vi "readAtom.vi"(4 "error in":errorcluster, 7 "Byte Stream File":refnum<file>) -> (0 "error out":errorcluster, 1 "String":string, 3 "Byte Stream File Refnum":refnum<file>)   [LabVIEW 2010]
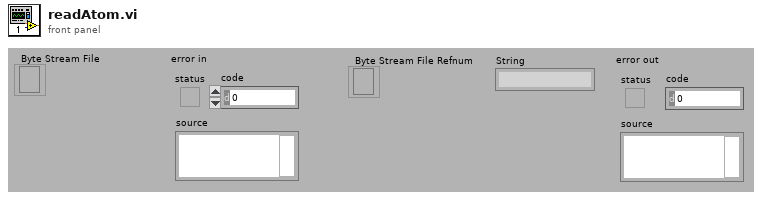
[diagram p1: front panel]
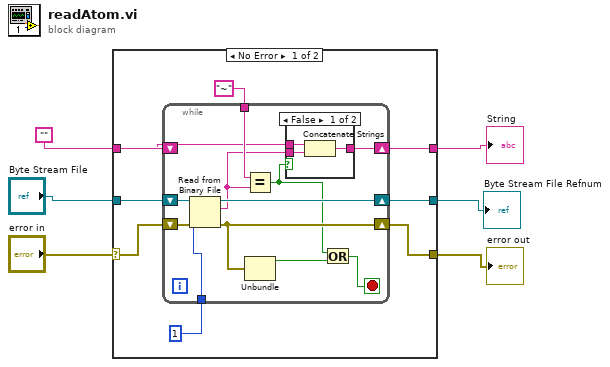
[diagram p0: block diagram]
diagram:
  n1 = case shown="No Error" "error in" {
    selector: "error in" -> [w12 w31]
    tunnel: "Byte Stream File" -> [w11 w32]
    tunnel: "" -> [w10 w33]
    tunnel: [w9 w33] -> w3
    tunnel: [w8 w32] -> w2
    tunnel: [w7 w31] -> w1
    frame No Error {
      n2 = while {
        shift-right: [w19] -> w9
        shift-left: w10 -> [w18]
        tunnel: "~" ("x") -> [w26]
        shift-right: [w25] -> w8
        shift-left: w11 -> [w24]
        shift-right: [w17] -> w7
        shift-left: w12 -> [w21]
        tunnel: 1 ("count") -> [w16]
        stop <- w22 stop-if-true
        n3 = Read from Binary File(8:w21, 10:w16, 11:w24) -> (0:w17:errorcluster, 2:w20:string, 3:w25:refnum<file>)  [unwired: 3 in, 1 out]
        n4 = Equal?(x=w26, y=w20) -> (x = y?=w15:bool)
        n5 = Unbundle(w17) -> ("status"=w23:bool)  [unwired: 2 out]
        n6 = case shown="False" w15 {
          tunnel: w20 -> [w29 _]
          tunnel: [w28 w30] -> w19
          tunnel: w18 -> [w27 w30]
          frame False {
            n7 = Concatenate Strings(w27, w29) -> (w28:string)
          }
          frame True {
          }
        }
        n8 = Or(x=w15, y=w23) -> (x .or. y?=w22:bool)
      }
    }
    frame Error {
    }
  }
  "Byte Stream File Refnum" <- w2
  "error out" <- w1
  "String" <- w3
